vi "CHECK MAST SAFETY.vi"(6 "PARAMETERS":T5={"MAST TOP"={"Descr"="", "Installed?"=FALSE, "A Channel"=enum."DIO 1", "Normally Closed?"=FALSE, "RefName"="", "stack name"=""}, "MAST BTM"={"Descr"="", "Installed?"=FALSE, "A Channel"=enum."DIO 1", "Normally Closed?"=FALSE, "RefName"="", "stack name"=""}, "SHUTTLE TOP"={"Descr"="", "Installed?"=FALSE, "A Channel"=enum."DIO 1", "Normally Closed?"=FALSE, "RefName"="", "stack name"=""}, "SHUTTLE BTM"={"Descr"="", "Installed?"=FALSE, "A Channel"=enum."DIO 1", "Normally Closed?"=FALSE, "RefName"="", "stack name"=""}, "ENCODER"={"Descr"="", "Installed?"=FALSE, "A Channel"=enum."DIO 1", "B Channel"=enum."DIO 1", "Invert Direction"=FALSE, "Enum"=enum."4x", "Gear ratio"=1.0, "Cycles per Rev"=360.0, "Diameter (in)"=0.15239999999999998, "RefName"="", "stack name"="", "min rate (hz)"=20.0, "Samples"=2, "STACK subnames"={"RESET name"="/reset", "STOPPED name"="/stopped", "DIRECTION name"="/direction", "RATE name"="/rate", "INSTALLED name"="/installed"}}, "TOP LIMIT stack name"="", "BTM LIMIT stack name"="", "Switches in series?"=FALSE}, 8 "error in (no error)":errorcluster, 9 "hold value":dbl, 11 "LIFT INPUT":dbl min=-1.0 max=1.0 step=0.1 format="%#_13g") -> (0 "error out":errorcluster, 1 "BTM LIMIT":bool, 2 "TOP LIMIT":bool, 3 "LIFT OUTPUT":dbl)   [LabVIEW 2018]
uses:
  Controls/def LIMIT SWITCH info.ctl
  <vilib>/Rock Robotics/SystemInterfaces/DIO/FPGA_DIOChannel.ctl
  Controls/def ENCODER info.ctl
  <vilib>/Rock Robotics/WPI/Encoder/WPI_EncoderType.ctl
  <vilib>/Rock Robotics/Network Tables/NT Write Boolean.vi
  <vilib>/Rock Robotics/Network Tables/NT Write Number.vi
panel:
  out "in series?":bool
  out "BTM MAST":bool
  out "BTM SHUTTLE":bool
  out "TOP SHUTTLE":bool
  out "TOP MAST":bool
  in  "stationary BTM":bool
  in  "shuttle BTM":bool
  in  "shuttle TOP":bool
  in  "stationary TOP":bool
  in  "stop":bool
  in  "testing?":bool
  # "STATUS & INPUT"
  # "OUTPUT"
  # "for TESTING ONLY"
  # "This function modifies the lift motor commands with respect to the mast limit switches.\n\nIF motor movement is up and both upper limit switches are active then the motor is forced to the HOLD VALUE and TOP LIMIT value is set to TRUE. \n\nIF motor movement is down and both lower limit switches are active then the motor is forced to the -HOLD VALUE and BTM LIMIT value is set to TRUE.  The encoder is also resest.\n\nALL limit switch ststus values and limit flags are written to the stack.\n\nMAST MOTOR value output & TOP/BTM limits are output directly.\n\nuse \"Switches in series?\" if the MAST and SHUTTLE limit switches are wired in series to create one TOP and one BTM circuit only; pgm will read/write values to the MAST TOP and BTM variables.\n\nNOTE: limit switches to DIO must be wired ground-signal, NOT +5V"
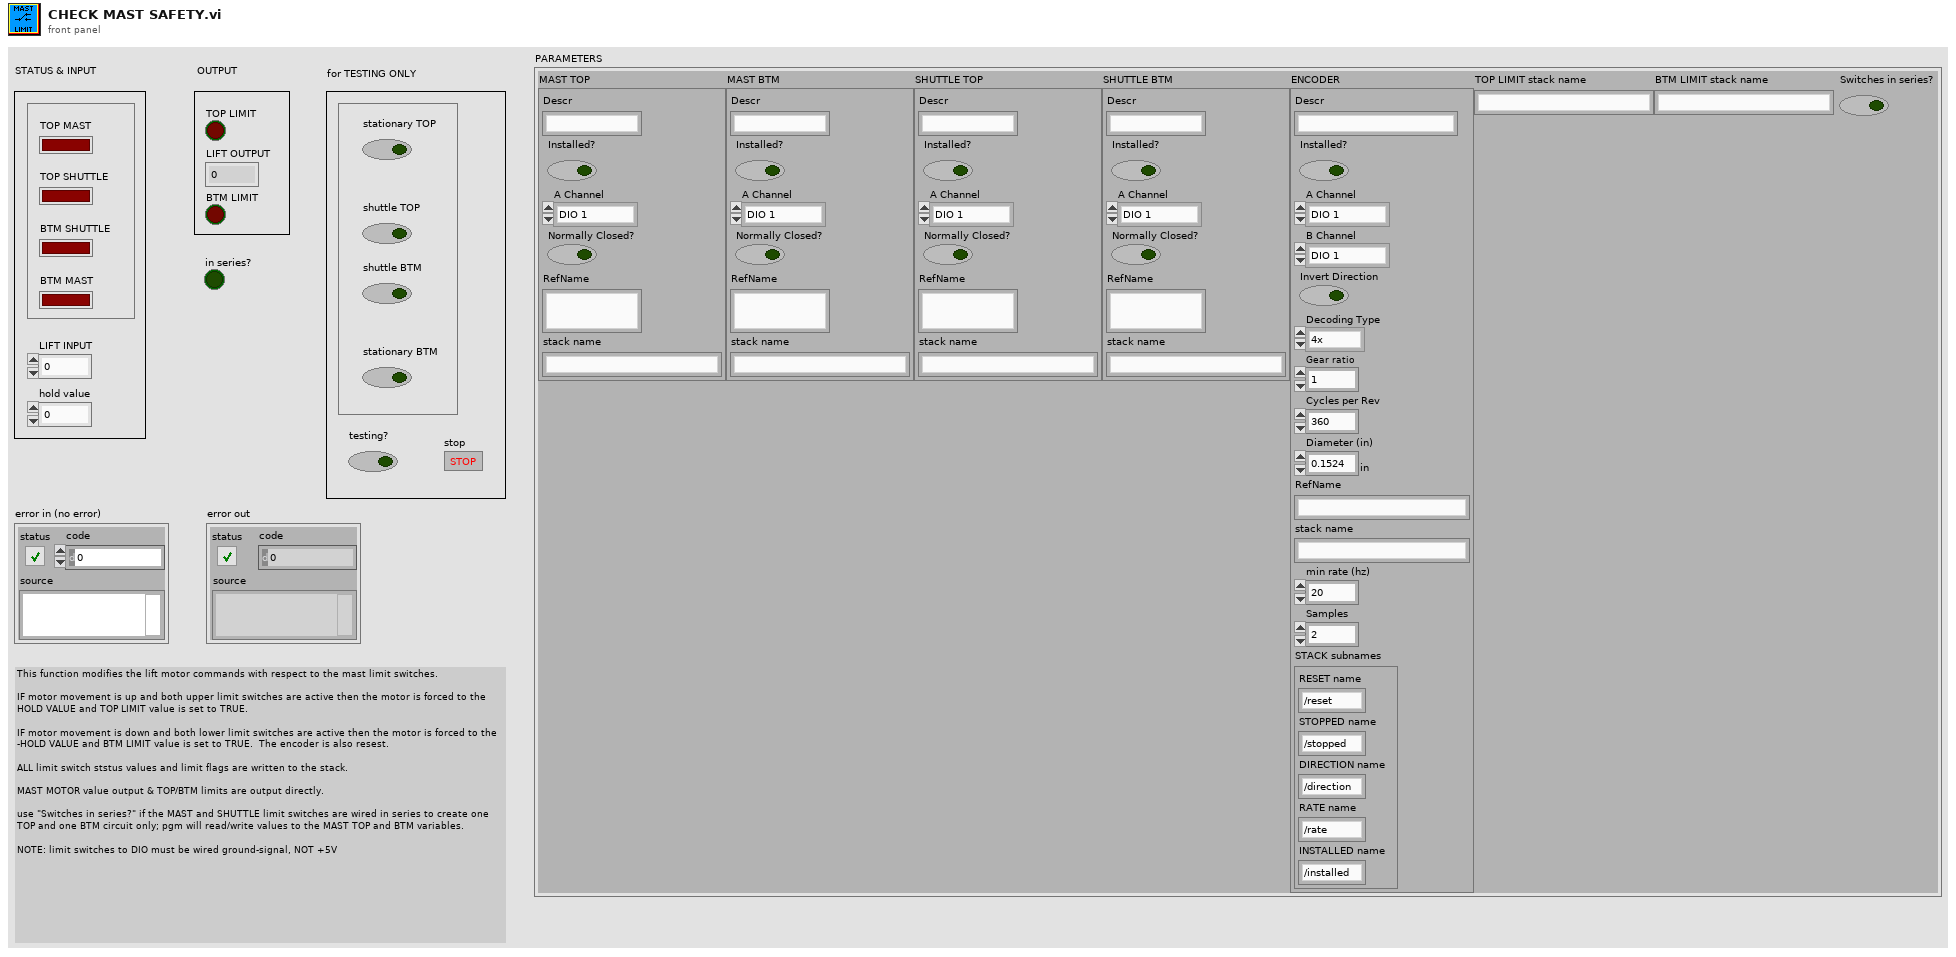
[diagram p1: front panel]
types:
  T1 = typedef "def LIMIT SWITCH info.ctl" = cluster{"Descr":string, "Installed?":bool, "A Channel":T2, "Normally Closed?":bool, "RefName":string, "stack name":string}
  T2 = typedef "FPGA_DIOChannel.ctl" = enum8{"DIO 0", "DIO 1", "DIO 2", "DIO 3", "DIO 4", "DIO 5", "DIO 6", "DIO 7", "DIO 8", "DIO 9", "DIO MXP 0", "DIO MXP 1", "DIO MXP 2", "DIO MXP 3", "DIO MXP 4", "DIO MXP 5", "DIO MXP 6", "DIO MXP 7", "DIO MXP 8", "DIO MXP 9", "DIO MXP 10", "DIO MXP 11", "DIO MXP 12", "DIO MXP 13", "DIO MXP 14", "DIO MXP 15", "SPI Port CS1", "SPI Port CS2", "SPI Port CS3", "SPI Port MISO", "SPI Port MOSI", "Invalid"}
  T3 = typedef "def ENCODER info.ctl" = cluster{"Descr":string, "Installed?":bool, "A Channel":T2, "B Channel":T2, "Invert Direction":bool, "Enum":T4, "Gear ratio":dbl, "Cycles per Rev":dbl, "Diameter (in)":dbl[unit], "RefName":string, "stack name":string, "min rate (hz)":dbl, "Samples":u8, "STACK subnames":cluster{"RESET name":string, "STOPPED name":string, "DIRECTION name":string, "RATE name":string, "INSTALLED name":string}}
  T4 = typedef "WPI_EncoderType.ctl" = enum16{"1x", "2x", "4x"}
  T5 = cluster{"MAST TOP":T1, "MAST BTM":T1, "SHUTTLE TOP":T1, "SHUTTLE BTM":T1, "ENCODER":T3, "TOP LIMIT stack name":string, "BTM LIMIT stack name":string, "Switches in series?":bool}
  T6 = typedef "WPI_SwitchDevRef.ctl" = cluster{"DevStatus":errorcluster, "DIO Channel":T2, "CntIndex":T7, "Normally Closed":bool}
  T7 = typedef "FPGA_CounterCtrSystemIndex.ctl" = enum8{"Ctr 0", "Ctr 1", "Ctr 2", "Ctr 3", "Ctr 4", "Ctr 5", "Ctr 6", "Ctr 7", "Invalid"}
  T8 = cluster{"stationary TOP":bool, "shuttle TOP":bool, "shuttle BTM":bool, "stationary BTM":bool}
  T9 = typedef "WPI_EncoderDevRef.ctl" = cluster{"DevStatus":errorcluster, "EncoderIndex":T10, "CounterIndex":T7, "DistancePerCount":dbl, "Decoding Type":T4}
  T10 = typedef "FPGA_EncoderIdx.ctl" = enum8{"Enc 0", "Enc 1", "Enc 2", "Enc 3", "Enc 4", "Enc 5", "Enc 6", "Enc 7", "Invalid"}
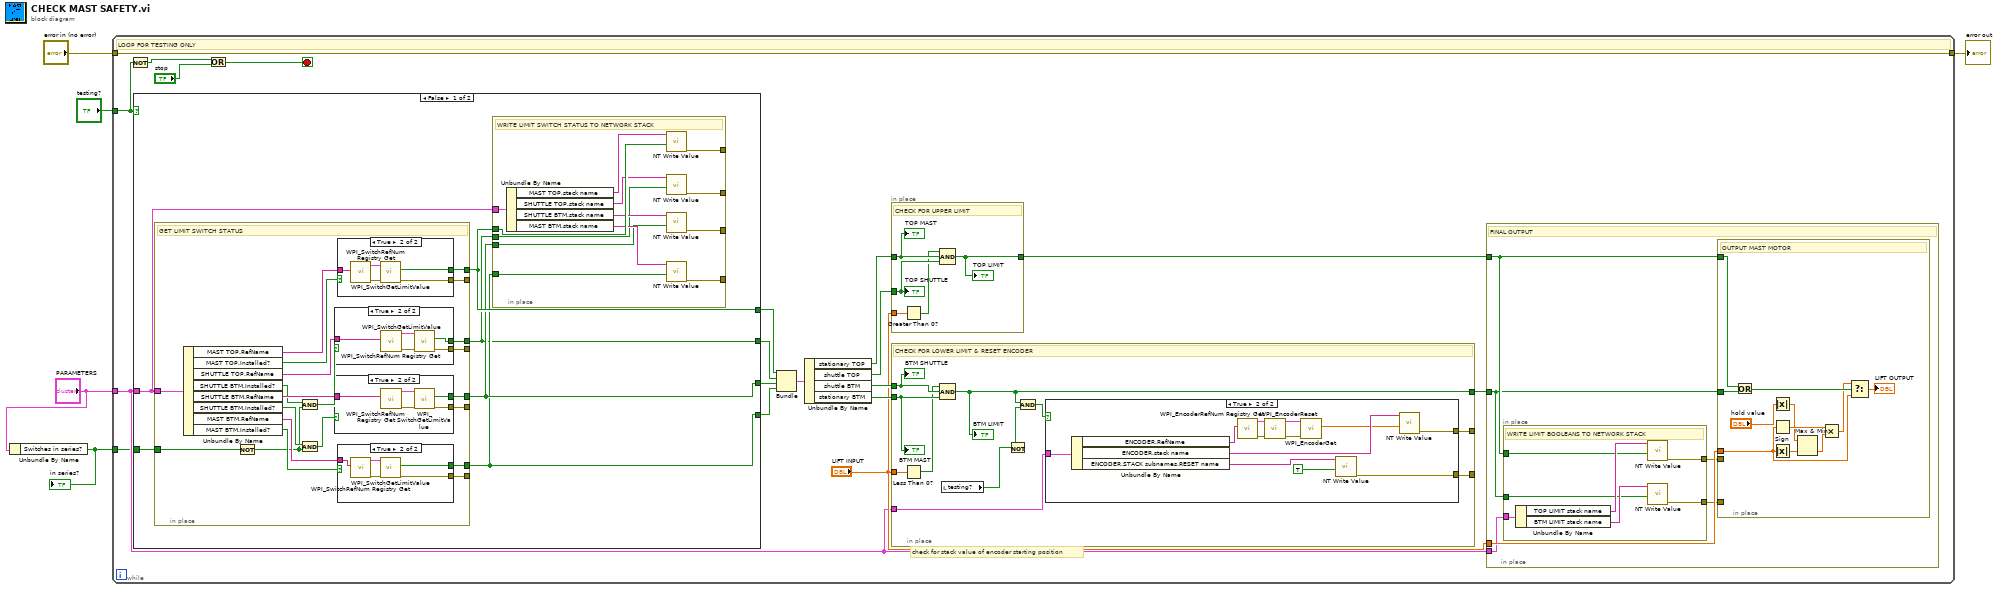
[diagram p0: block diagram]
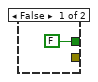
[diagram p3: hidden frame]
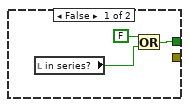
[diagram p4: hidden frame]
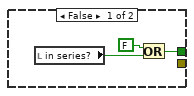
[diagram p5: hidden frame]
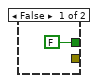
[diagram p6: hidden frame]
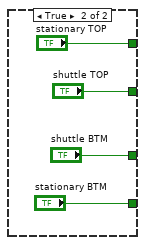
[diagram p7: hidden frame]
diagram:
  n1 = Unbundle By Name("PARAMETERS") -> ("Switches in series?"=w1:bool)
  "in series?" <- w1
  n2 = while {
    tunnel: "testing?" -> [w17]
    tunnel: [w10] -> w4
    tunnel: "error in (no error)" -> [w10]
    tunnel: "PARAMETERS" -> [w9]
    tunnel: w1 -> [w6]
    stop <- w23 stop-if-true
    # "check for stack value of encoder starting position"
    # "LOOP FOR TESTING ONLY"
    n3 = Not(x=w17) -> (.not. x?=w22:bool)
    n4 = case shown="False" w17 {
      tunnel: [w81 "stationary TOP"] -> w16
      tunnel: [w78 "shuttle TOP"] -> w15
      tunnel: [w80 "shuttle BTM"] -> w14
      tunnel: [w79 "stationary BTM"] -> w13
      tunnel: w9 -> [w82 _]
      tunnel: w6 -> [w77 _]
      frame False {
        n5 = in-place {
          in-place-border: [w116] -> w79
          in-place-border: [w115] -> w80
          in-place-border: [w114] -> w78
          in-place-border: [w113] -> w81
          in-place-border: w82 -> [w111]
          in-place-border: [w110] -> _
          in-place-border: [w109] -> _
          in-place-border: [w108] -> _
          in-place-border: [w107] -> _
          in-place-border: w77 -> [w97]
          # "GET LIMIT SWITCH STATUS"
          n6 = Unbundle By Name(w111) -> ("MAST TOP.RefName"=w112:string, "MAST TOP.Installed?"=w105:bool, "SHUTTLE TOP.RefName"=w106:string, "SHUTTLE BTM.Installed?"=w100:bool, "SHUTTLE BTM.RefName"=w104:string, "SHUTTLE BTM.Installed?"=w101:bool, "MAST BTM.RefName"=w103:string, "MAST BTM.Installed?"=w102:bool)
          n7 = Not(x=w97) -> (.not. x?=w96:bool)
          n8 = And(x=w100, y=w96) -> (x .and. y?=w99:bool)
          n9 = And(x=w101, y=w96) -> (x .and. y?=w98:bool)
          n10 = case shown="True" w99 {
            tunnel: [w132 w136] -> w114
            tunnel: w106 -> [_ w135]
            tunnel: [_ w134] -> w109
            frame False {
              n11 = local read "in series?"() -> (w131:bool)
              n12 = Or(x=FALSE, y=w131) -> (x .or. y?=w132:bool)
            }
            frame True {
              n13 = call <vilib>:"WPI_SwitchRefNum Registry Get.vi"("refnum name"=w135) -> ("error out"=w138:errorcluster, "SwitchDevRef"=w137:T6)  [unwired: 9 in]
              n14 = call <vilib>:"WPI_SwitchGetLimitValue.vi"("error in (no error)"=w138, "SwitchDevRef"=w137) -> ("error out"=w134:errorcluster, "Switch Pressed"=w136:bool)  [unwired: 7 in, 1 out]
            }
          }
          n15 = case shown="True" w98 {
            tunnel: [w125 w128] -> w115
            tunnel: w104 -> [_ w127]
            tunnel: [_ w126] -> w108
            frame False {
              n16 = local read "in series?"() -> (w123:bool)
              n17 = Or(x=FALSE, y=w123) -> (x .or. y?=w125:bool)
            }
            frame True {
              n18 = call <vilib>:"WPI_SwitchRefNum Registry Get.vi"("refnum name"=w127) -> ("error out"=w130:errorcluster, "SwitchDevRef"=w129:T6)  [unwired: 9 in]
              n19 = call <vilib>:"WPI_SwitchGetLimitValue.vi"("error in (no error)"=w130, "SwitchDevRef"=w129) -> ("error out"=w126:errorcluster, "Switch Pressed"=w128:bool)  [unwired: 7 in, 1 out]
            }
          }
          n20 = case shown="True" w105 {
            tunnel: [FALSE w142] -> w113
            tunnel: w112 -> [_ w141]
            tunnel: [_ w140] -> w110
            frame False {
            }
            frame True {
              n21 = call <vilib>:"WPI_SwitchRefNum Registry Get.vi"("refnum name"=w141) -> ("error out"=w144:errorcluster, "SwitchDevRef"=w143:T6)  [unwired: 9 in]
              n22 = call <vilib>:"WPI_SwitchGetLimitValue.vi"("error in (no error)"=w144, "SwitchDevRef"=w143) -> ("error out"=w140:errorcluster, "Switch Pressed"=w142:bool)  [unwired: 7 in, 1 out]
            }
          }
          n23 = case shown="True" w102 {
            tunnel: [FALSE w120] -> w116
            tunnel: w103 -> [_ w119]
            tunnel: [_ w118] -> w107
            frame False {
            }
            frame True {
              n24 = call <vilib>:"WPI_SwitchRefNum Registry Get.vi"("refnum name"=w119) -> ("error out"=w122:errorcluster, "SwitchDevRef"=w121:T6)  [unwired: 9 in]
              n25 = call <vilib>:"WPI_SwitchGetLimitValue.vi"("error in (no error)"=w122, "SwitchDevRef"=w121) -> ("error out"=w118:errorcluster, "Switch Pressed"=w120:bool)  [unwired: 7 in, 1 out]
            }
          }
        }
        n26 = in-place {
          in-place-border: w82 -> [w95]
          in-place-border: w81 -> [w93]
          in-place-border: w80 -> [w89]
          in-place-border: w79 -> [w88]
          in-place-border: w78 -> [w87]
          in-place-border: [w86] -> _
          in-place-border: [w85] -> _
          in-place-border: [w84] -> _
          in-place-border: [w83] -> _
          # "WRITE LIMIT SWITCH STATUS TO NETWORK STACK"
          n27 = Unbundle By Name(w95) -> ("MAST TOP.stack name"=w94:string, "SHUTTLE TOP.stack name"=w91:string, "SHUTTLE BTM.stack name"=w90:string, "MAST BTM.stack name"=w92:string)
          n28 = call-poly <vilib>:"NT Write Value.vi"("Boolean"=w93, "Name"=w94) -> ("error out"=w86:errorcluster)  [unwired: 9 in]
          n29 = call-poly <vilib>:"NT Write Value.vi"("Boolean"=w87, "Name"=w91) -> ("error out"=w85:errorcluster)  [unwired: 9 in]
          n30 = call-poly <vilib>:"NT Write Value.vi"("Boolean"=w89, "Name"=w90) -> ("error out"=w84:errorcluster)  [unwired: 9 in]
          n31 = call-poly <vilib>:"NT Write Value.vi"("Boolean"=w88, "Name"=w92) -> ("error out"=w83:errorcluster)  [unwired: 9 in]
        }
      }
      frame True {
      }
    }
    n32 = Or(x=w22, y="stop") -> (x .or. y?=w23:bool)
    n33 = Bundle("stationary TOP"=w16, "shuttle TOP"=w15, "shuttle BTM"=w14, "stationary BTM"=w13) -> (w12:T8)  [unwired: 1 in]
    n34 = Unbundle By Name(w12) -> ("stationary TOP"=w21:bool, "shuttle TOP"=w20:bool, "shuttle BTM"=w19:bool, "stationary BTM"=w18:bool)
    n35 = in-place {
      in-place-border: w21 -> [w76]
      in-place-border: w20 -> [w75]
      in-place-border: "LIFT INPUT" -> [w74]
      in-place-border: [w72] -> w8
      # "CHECK FOR UPPER LIMIT"
      n36 = Greater Than 0?(x=w74) -> (x > 0?=w73:bool)
      n37 = Compound Arithmetic op=AND(w73, w76, w75) -> (w72:bool)
      "TOP LIMIT" <- w72
      "TOP SHUTTLE" <- w75
      "TOP MAST" <- w76
    }
    n38 = in-place {
      in-place-border: w19 -> [w59]
      in-place-border: w18 -> [w58]
      in-place-border: "LIFT INPUT" -> [w57]
      in-place-border: [w56] -> w7
      in-place-border: w9 -> [w55]
      in-place-border: [w54] -> _
      in-place-border: [w53] -> _
      # "CHECK FOR LOWER LIMIT & RESET ENCODER"
      n39 = Less Than 0?(x=w57) -> (x < 0?=w52:bool)
      n40 = Compound Arithmetic op=AND(w52, w59, w58) -> (w56:bool)
      "BTM LIMIT" <- w56
      n41 = local read "testing?"() -> (w50:bool)
      n42 = Not(x=w50) -> (.not. x?=w49:bool)
      n43 = And(x=w56, y=w49) -> (x .and. y?=w51:bool)
      n44 = case shown="True" w51 {
        tunnel: w55 -> [_ w71]
        tunnel: [_ w63] -> w54
        tunnel: [_ w60] -> w53
        frame False {
        }
        frame True {
          n45 = Unbundle By Name(w71) -> ("ENCODER.RefName"=w68:string, "ENCODER.stack name"=w65:string, "ENCODER.STACK subnames.RESET name"=w62:string)
          n46 = call <vilib>:"WPI_EncoderRefNum Registry Get.vi"("refnum name"=w68) -> ("error out"=w70:errorcluster, "EncoderDevRef"=w69:T9)  [unwired: 9 in]
          n47 = call <vilib>:"WPI_EncoderReset.vi"("error in (no error)"=w70, "EncoderDevRef"=w69) -> ("error out"=w67:errorcluster, "EncoderDevRef"=w66:T9)  [unwired: 8 in]
          n48 = call <vilib>:"WPI_EncoderGet.vi"("error in (no error)"=w67, "EncoderDevRef"=w66) -> ("Distance"=w64:dbl)  [unwired: 4 in, 5 out]
          n49 = call-poly <vilib>:"NT Write Value.vi"("Boolean"=TRUE, "Name"=w62) -> ("error out"=w60:errorcluster)  [unwired: 9 in]
          n50 = call-poly <vilib>:"NT Write Value.vi"("Numeric"=w64, "Name"=w65) -> ("error out"=w63:errorcluster)  [unwired: 9 in]
        }
      }
      "BTM SHUTTLE" <- w59
      "BTM MAST" <- w58
    }
    n51 = in-place {
      in-place-border: "LIFT INPUT" -> [w30]
      in-place-border: w9 -> [w29]
      in-place-border: w8 -> [w28]
      in-place-border: w7 -> [w27]
      # "FINAL OUTPUT"
      n52 = in-place {
        in-place-border: w29 -> [w37]
        in-place-border: w28 -> [w35]
        in-place-border: w27 -> [w33]
        in-place-border: [w32] -> w26
        in-place-border: [w31] -> w25
        # "WRITE LIMIT BOOLEANS TO NETWORK STACK"
        n53 = Unbundle By Name(w37) -> ("TOP LIMIT stack name"=w36:string, "BTM LIMIT stack name"=w34:string)
        n54 = call-poly <vilib>:"NT Write Value.vi"("Boolean"=w35, "Name"=w36) -> ("error out"=w32:errorcluster)  [unwired: 9 in]
        n55 = call-poly <vilib>:"NT Write Value.vi"("Boolean"=w33, "Name"=w34) -> ("error out"=w31:errorcluster)  [unwired: 9 in]
      }
      n56 = in-place {
        in-place-border: w27 -> [w48]
        in-place-border: w28 -> [w47]
        in-place-border: w30 -> [w40]
        in-place-border: w26 -> [_]
        in-place-border: w25 -> [_]
        # "OUTPUT MAST MOTOR"
        n57 = Or(x=w47, y=w48) -> (x .or. y?=w46:bool)
        n58 = Absolute Value(x="hold value") -> (abs(x)=w41:dbl)
        n59 = Sign(1:w40) -> (0:w42:dbl)
        n60 = Absolute Value(x=w40) -> (abs(x)=w39:dbl)
        n61 = Max & Min(x=w41, y=w39) -> (min(x,y)=w38:dbl)  [unwired: 1 out]
        n62 = Multiply(x=w42, y=w38) -> (x*y=w43:dbl)
        n63 = Select(t=w43, s=w46, f=w40) -> (s? t:f=→"LIFT OUTPUT":dbl)
      }
    }
  }
  "error out" <- w4
